vi "wrap_JointPositions.vi"(0 "Mode":enum16{"Position", "Velocity", "Effort"}(ring), 3 "Side":T1, 4 "Positions":dbl[](array[numeric]), 5 "msg in":string) -> (2 "msg out":string)   [LabVIEW 2013]
uses:
  Code/SubVIs/BaxterSide.ctl
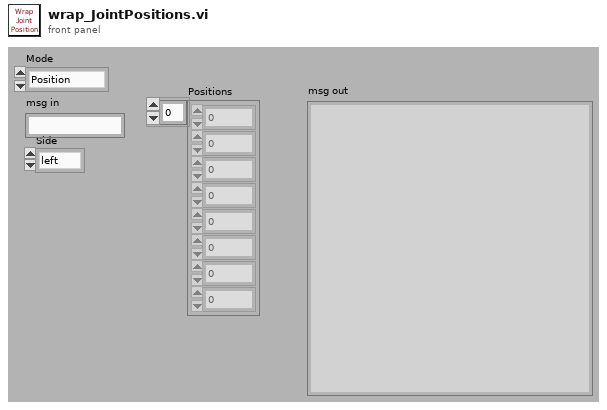
[diagram p1: front panel]
types:
  T1 = typedef "BaxterSide.ctl" = enum16{"left", "right"}
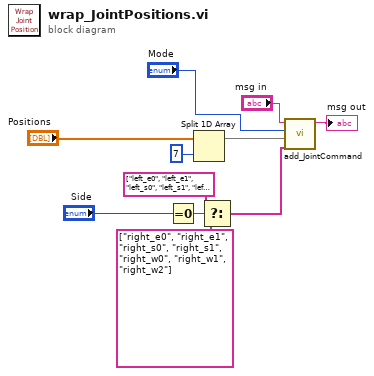
[diagram p0: block diagram]
diagram:
  n1 = Equal To 0?(x="Side") -> (x = 0?=w10:bool)
  n2 = Split 1D Array(array="Positions", index=7) -> (first subarray=w4:dbl[])  [unwired: 1 out]
  n3 = Select(t=string[] ["left_e0", "left_e1", "left_s0", "left_s1", "left_w0", "left_w1", "left_w2"] ("left"), s=w10, f=string[] ["right_e0", "right_e1", "right_s0", "right_s1", "right_w0", "right_w1", "right_w2"] ("right")) -> (s? t:f=w7:string[])
  n4 = call "add_JointCommand.vi"("Names"=w7, "Angles"=w4, "Mode"="Mode", "msg in"="msg in") -> ("msg out"=→"msg out":string)  [unwired: 3 in]
